vi "Connect EventReg Wire If not Connected.vi"(8 "error in (no error)":errorcluster, 10 "case":string, 11 "CSM-Helper in":refnum<class "CSM-Helper.lvclass">) -> (0 "error out":errorcluster, 3 "CSM-Helper out":refnum<class "CSM-Helper.lvclass">)   [LabVIEW 2017, in "CSM-Helper.lvclass"]
doc: "### Connect EventReg Wire If not Connected.vi\n\n-- <b>Controls</b> --\n- <b>case</b>:\n- <b>CSM-Helper in</b>: CSMHelper input\n\n-- <b>Indicators</b> --\n- <b>CSM-Helper out</b>: CSMHelper output"
uses:
  CSM-Helper.lvclass
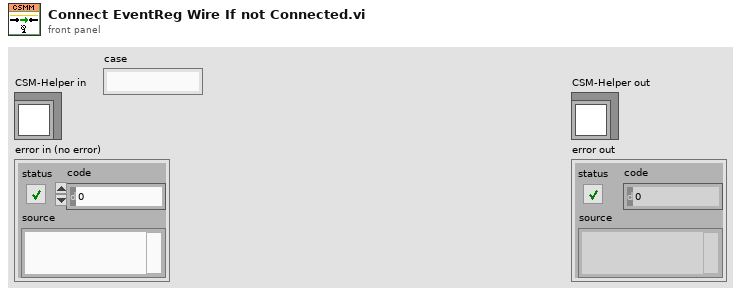
[diagram p1: front panel]
types:
  T1 = cluster{"Registration":refnum<vi>, "InternalData":refnum<vi>, "CSM Name":refnum<vi>, "Last Resp":refnum<vi>, "Remaining State":refnum<vi>, "Arguments":refnum<vi>, "Response Source":refnum<vi>, "Source CSM":refnum<vi>, "Selector":refnum<vi>, "Error":refnum<vi>}
  T2 = cluster{"Registration":refnum<vi>, "InternalData":refnum<vi>, "Resp":refnum<vi>, "Remaining State":refnum<vi>, "Error":refnum<vi>}
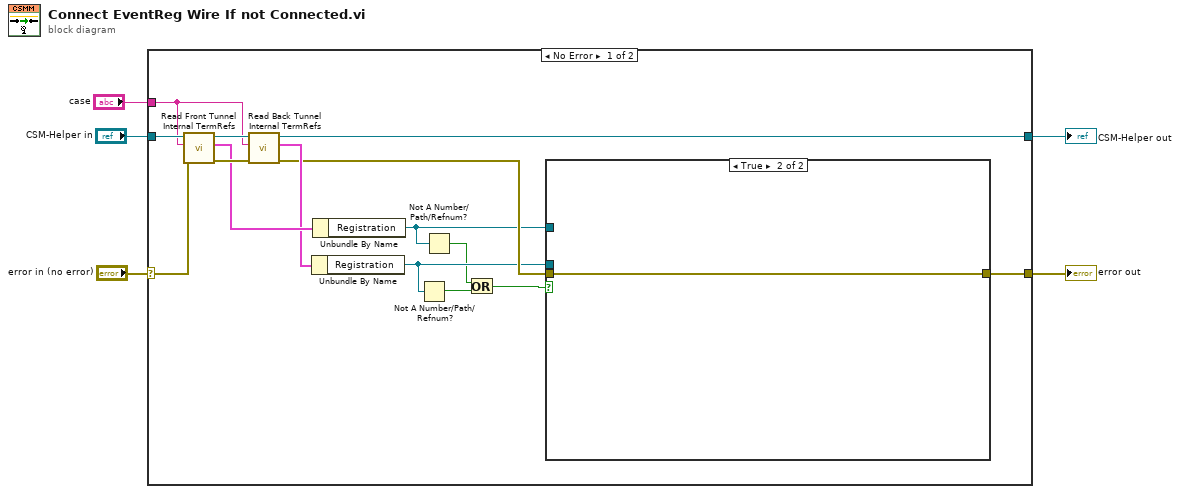
[diagram p0: block diagram]
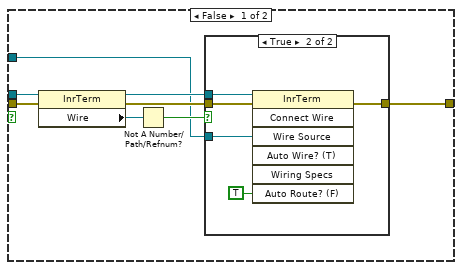
[diagram p2: hidden frame]
diagram:
  n1 = case shown="No Error" "error in (no error)" {
    selector: "error in (no error)" -> [w13 w37]
    tunnel: "CSM-Helper in" -> [w15 w36]
    tunnel: [w14 w36] -> w4
    tunnel: [w12 w37] -> w2
    tunnel: "case" -> [w11 _]
    frame No Error {
      n2 = call "Read Front Tunnel Internal TermRefs.vi"("error in (no error)"=w13, "case"=w11, "CSM-Helper in"=w15) -> ("error out"=w19:errorcluster, "Front Tunnels"=w18:T1, "CSM-Helper out"=w20:refnum<class "CSM-Helper.lvclass">)  [unwired: 6 in]
      n3 = call "Read Back Tunnel Internal TermRefs.vi"("error in (no error)"=w19, "element"=w11, "CSM-Helper in"=w20) -> ("error out"=w16:errorcluster, "Back Tunnels"=w17:T2, "CSM-Helper out"=w14:refnum<class "CSM-Helper.lvclass">)  [unwired: 6 in]
      n4 = Unbundle By Name(w17) -> ("Registration"=w10:refnum<vi>)
      n5 = Unbundle By Name(w18) -> ("Registration"=w9:refnum<vi>)
      n6 = Not A Number/Path/Refnum?(number/path/refnum=w10) -> (NaN/Path/Refnum?=w8:bool)
      n7 = Not A Number/Path/Refnum?(number/path/refnum=w9) -> (NaN/Path/Refnum?=w7:bool)
      n8 = Or(x=w7, y=w8) -> (x .or. y?=w6:bool)
      n9 = case shown="True" w6 {
        tunnel: w16 -> [w24 w35]
        tunnel: [w23 w35] -> w12
        tunnel: w10 -> [w22 _]
        tunnel: w9 -> [w21 _]
        frame False {
          n10 = property class="InrTerm"(reference=w22, error in=w24) -> (reference out=w27:refnum<vi>, error out=w25:errorcluster, "Wire"=w28:refnum<vi>)
          n11 = Not A Number/Path/Refnum?(number/path/refnum=w28) -> (NaN/Path/Refnum?=w26:bool)
          n12 = case shown="True" w26 {
            tunnel: w27 -> [_ w34]
            tunnel: w21 -> [_ w33]
            tunnel: w25 -> [w29 w31]
            tunnel: [w29 w30] -> w23
            frame False {
            }
            frame True {
              n13 = invoke class="InrTerm" method="Connect Wire"(reference=w34, error in=w31, "Wire Source"=w33, "Auto Route? (F)"=TRUE) -> (error out=w30:errorcluster)  [unwired: 3 in, 6 out]
            }
          }
        }
        frame True {
        }
      }
    }
    frame Error {
    }
  }
  "CSM-Helper out" <- w4
  "error out" <- w2
